vi "test_ring.vi"(9 "b":dbl, 10 "operator":u16(ring) items=["+", "*"], 11 "a":dbl) -> (3 "c":dbl)   [LabVIEW 2020]
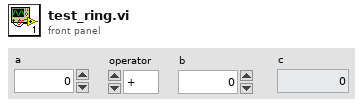
[diagram p1: front panel]
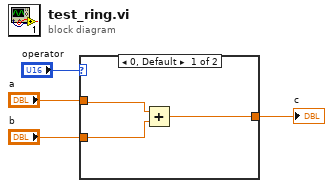
[diagram p0: block diagram]
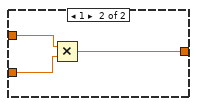
[diagram p2: hidden frame]
diagram:
  n1 = case shown="0, Default" "operator" {
    tunnel: "a" -> [w7 w10]
    tunnel: "b" -> [w6 w9]
    tunnel: [w5 w8] -> w1
    frame 0, Default {
      n2 = Add(x=w7, y=w6) -> (x+y=w5:dbl)
    }
    frame 1 {
      n3 = Multiply(x=w10, y=w9) -> (x*y=w8:dbl)
    }
  }
  "c" <- w1
